vi "Find Structures.vi"(8 "error in (no error)":errorcluster, 9 "i in":i32, 11 "VI in":refnum<vi>) -> (0 "error out":errorcluster, 1 "i out":i32, 3 "Structures":T1[](array[typedef]))   [LabVIEW 2023, in "VIDoc Parsing.lvlib" / "Structure Reporter.lvlib"]
uses:
  Structure Reporter.lvlib
  Structure Result 2.ctl
  <vilib>/Utility/traverseref.llb/TRef TravTarget.ctl
  <vilib>/Utility/traverseref.llb/VI Scripting - Traverse.lvlib
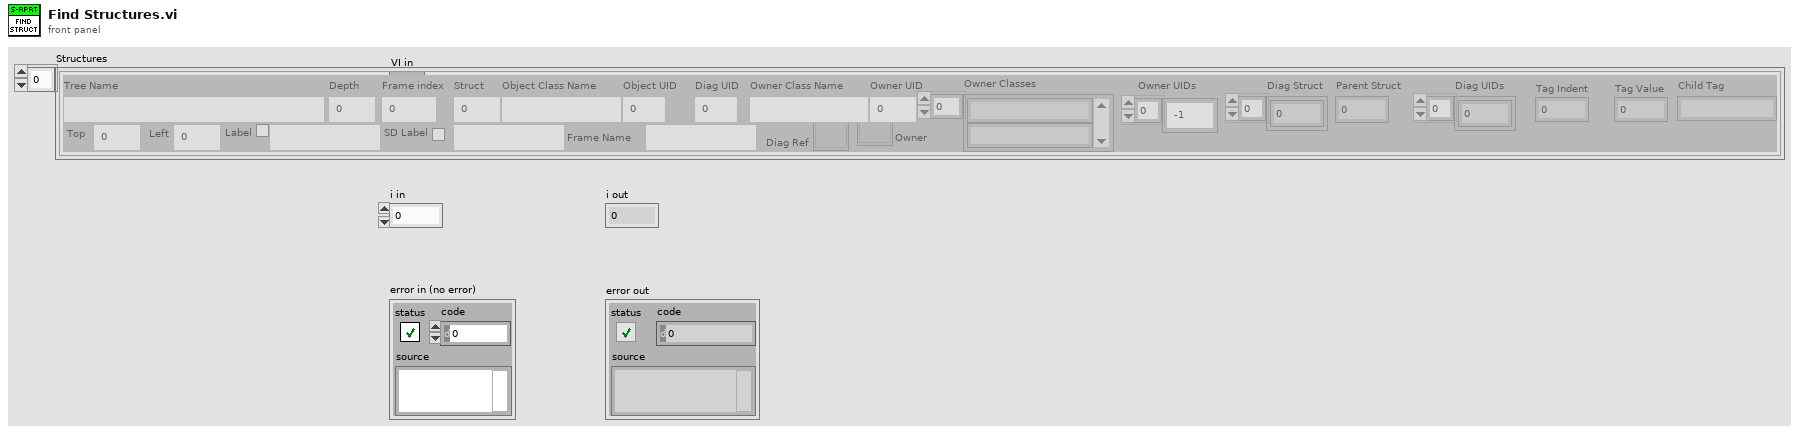
[diagram p1: front panel]
types:
  T1 = typedef "VIDoc Parsing.lvlib/Structure Reporter.lvlib/Structure Result 2.ctl" = cluster{"Depth":i32, "Top":i32, "Left":i32, "Frame index":i32, "Struct":i32, "Object Class Name":string, "Object UID":i32, "Label Visible":bool, "Object Label":string, "SD Label Visible":bool, "Object SD Label":string, "Frame Name":string, "Diag UID":i32, "Owner Class Name":string, "Owner UID":i32, "Diag Struct":i32[], "Parent Struct":i32, "Diag UIDs":i32[], "Tree Name":string, "Diag Ref":refnum<vi>, "Owner Classes":string[], "Owner":refnum<vi>, "Owner UIDs":i32[], "Tag Indent":i32, "Tag Value":i32, "Child Tag":string}
  T2 = typedef "TRef TravTarget.ctl" = enum16{"FP", "BD", "Other"}
  T3 = enum32{"Conditional Disable Style", "Diagram Disable Style", "Type Specialization Style"}
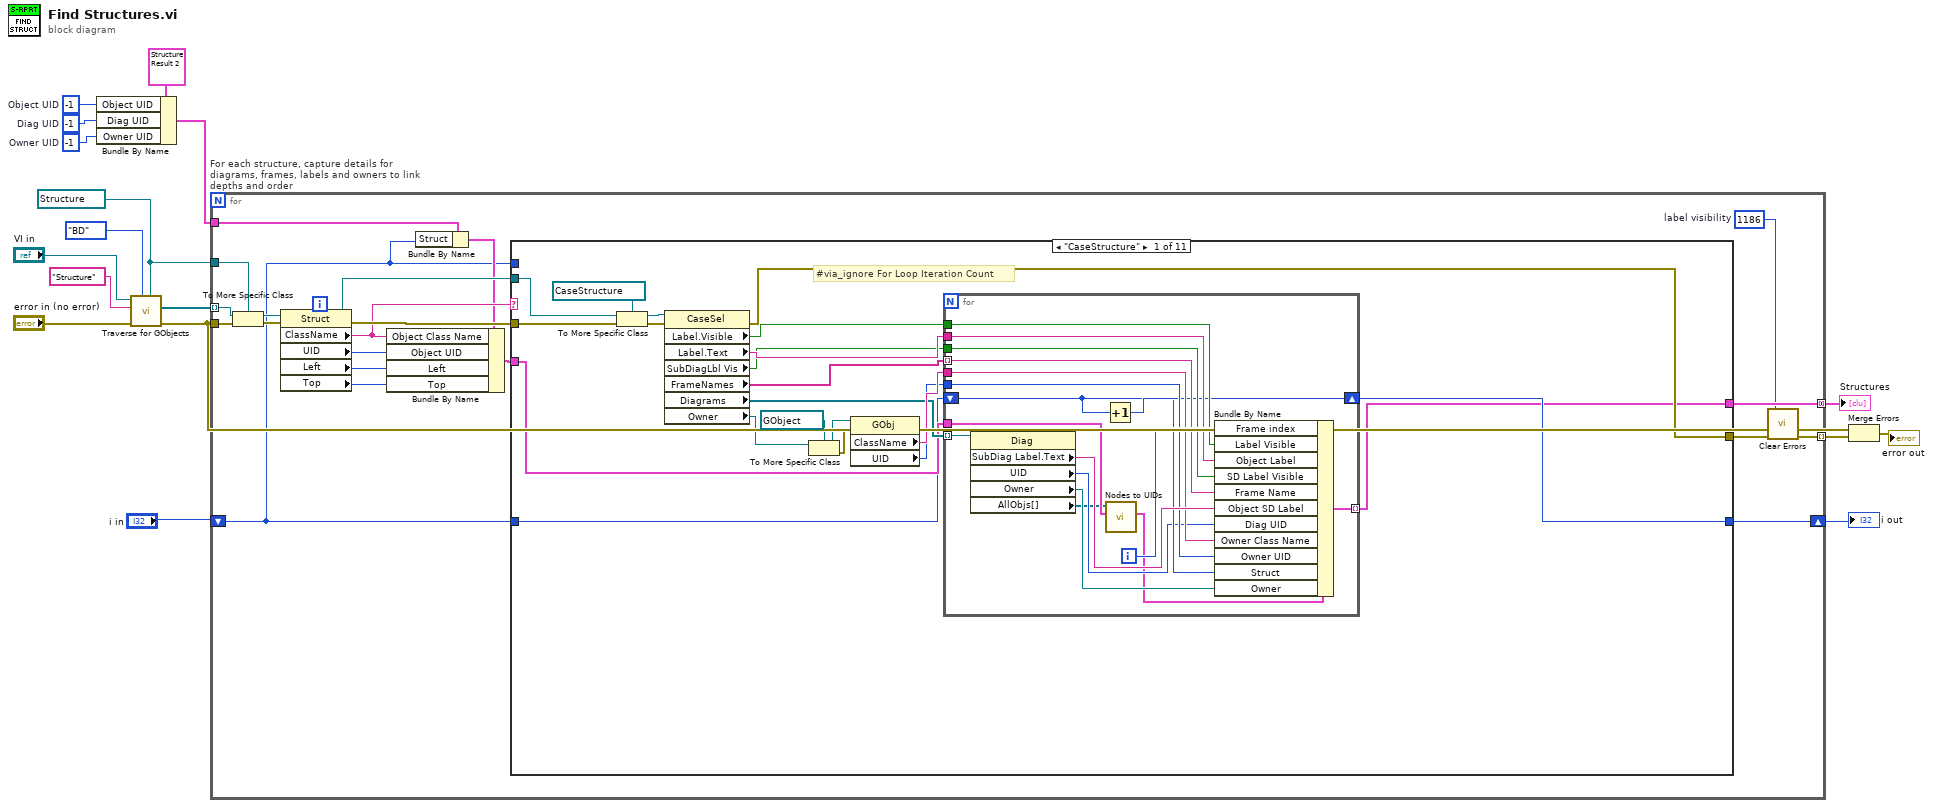
[diagram p0: block diagram]
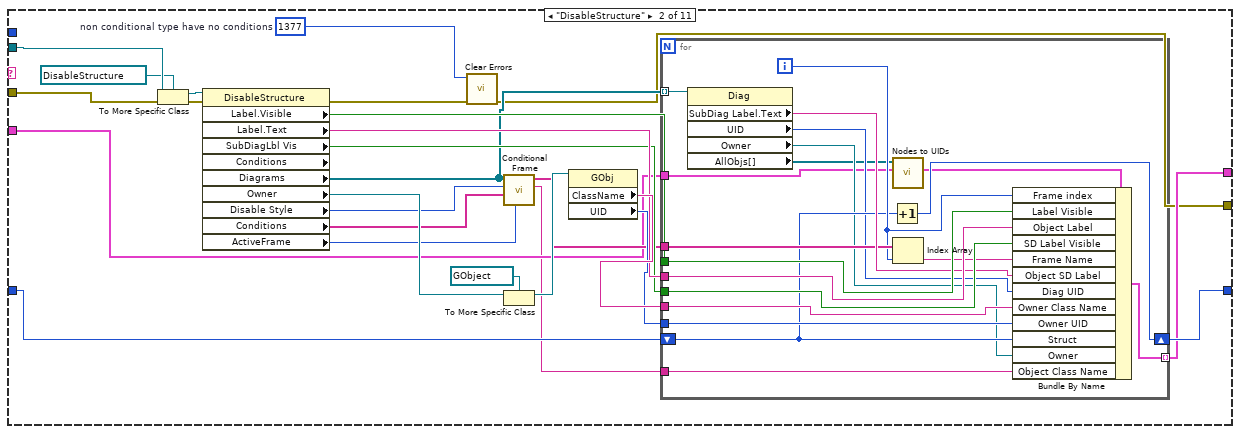
[diagram p2: hidden frame]
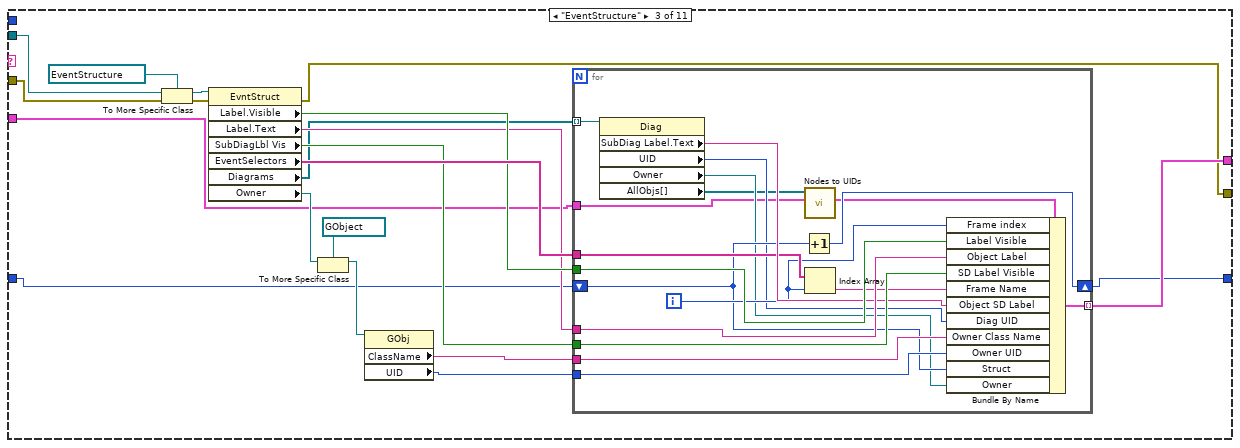
[diagram p3: hidden frame]
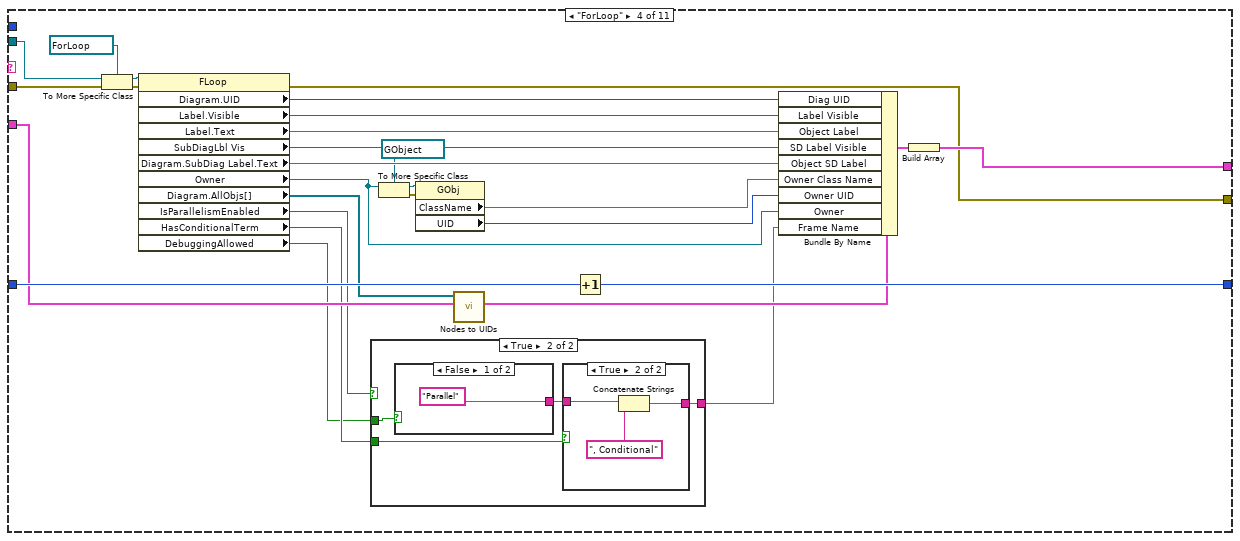
[diagram p4: hidden frame]
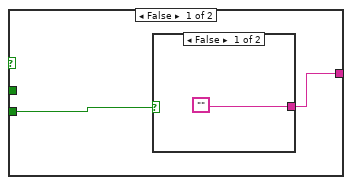
[diagram p5: hidden frame]
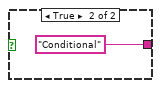
[diagram p6: hidden frame]
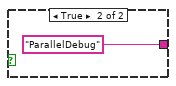
[diagram p8: hidden frame]
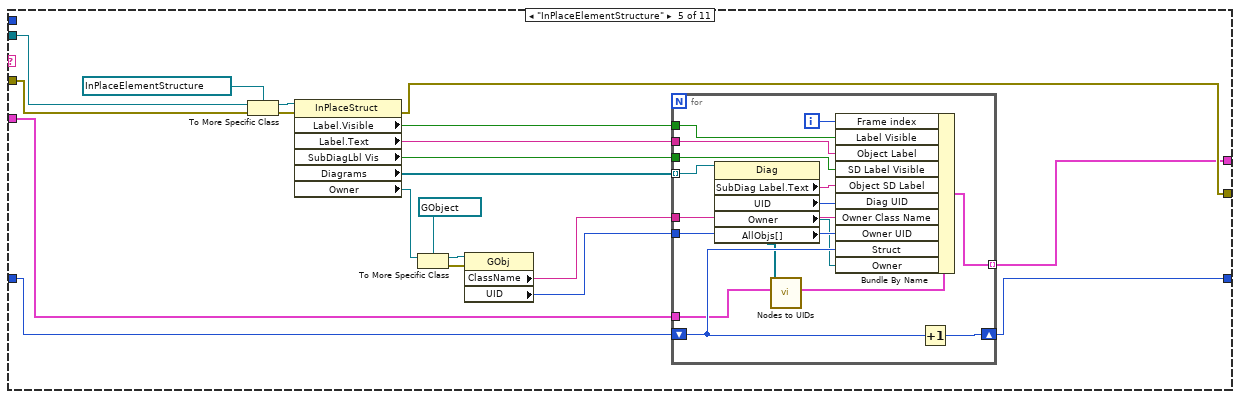
[diagram p9: hidden frame]
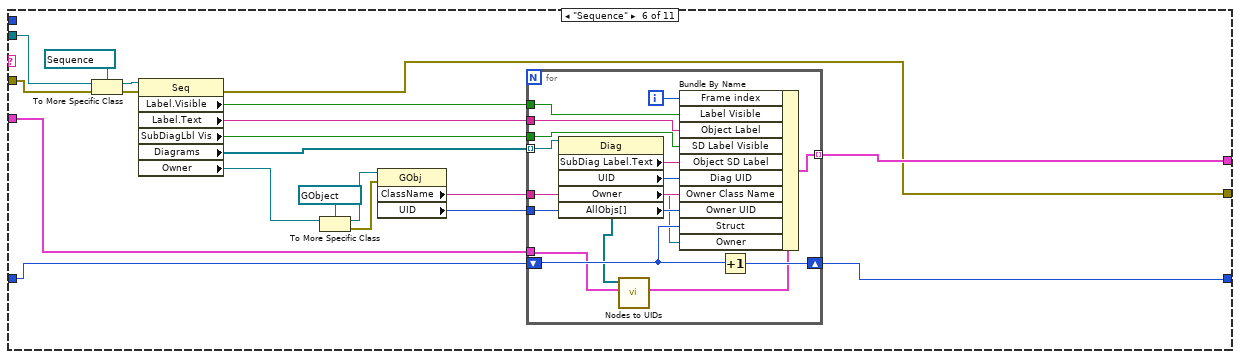
[diagram p10: hidden frame]
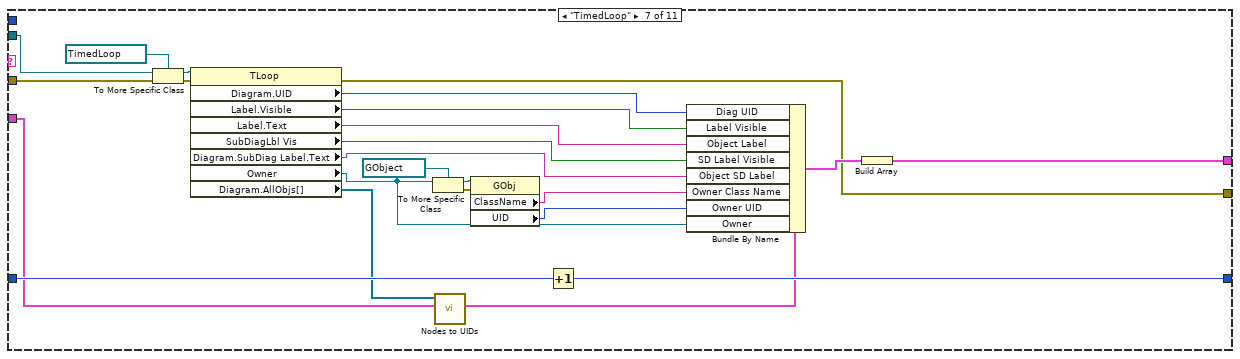
[diagram p11: hidden frame]
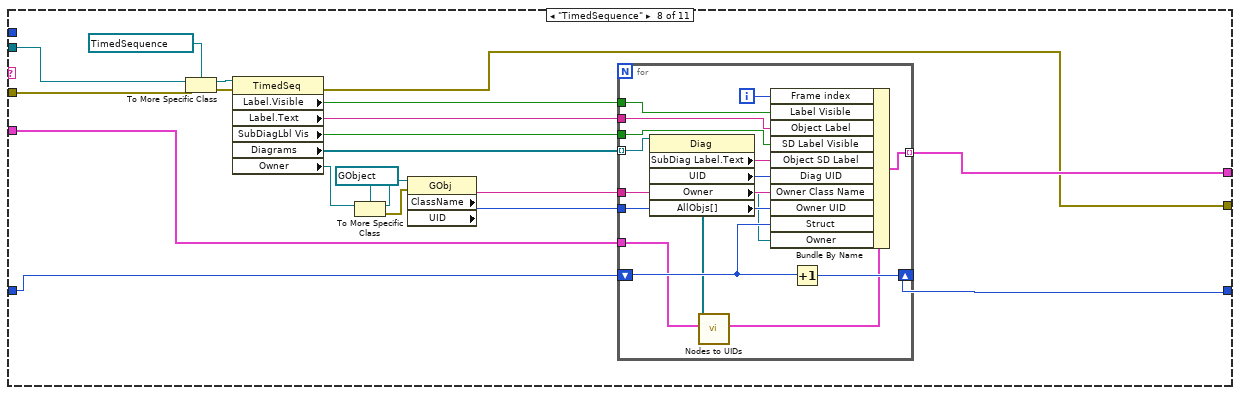
[diagram p12: hidden frame]
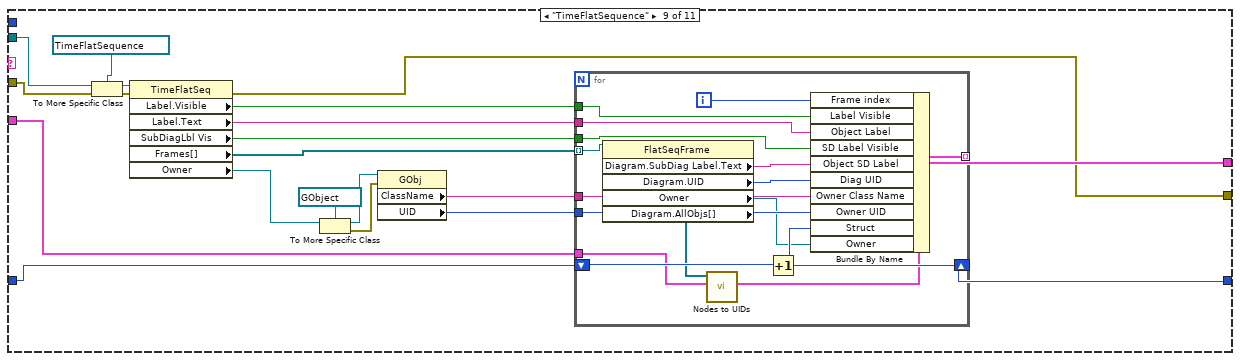
[diagram p13: hidden frame]
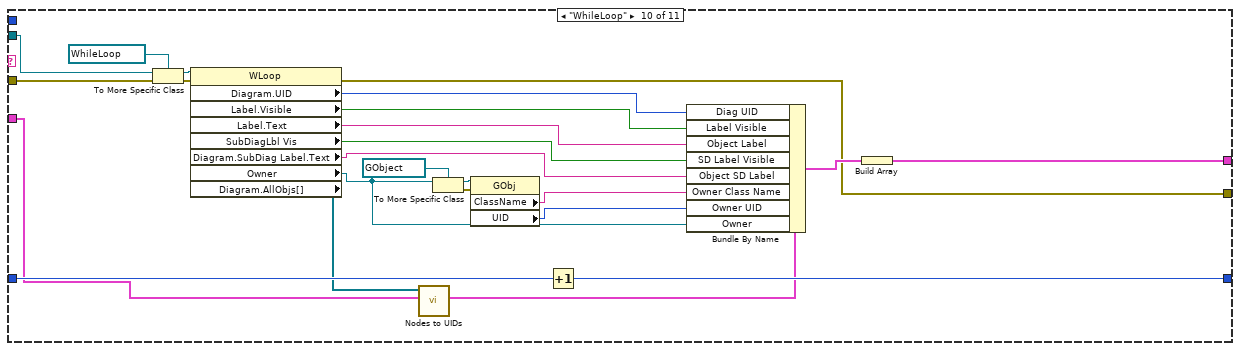
[diagram p14: hidden frame]
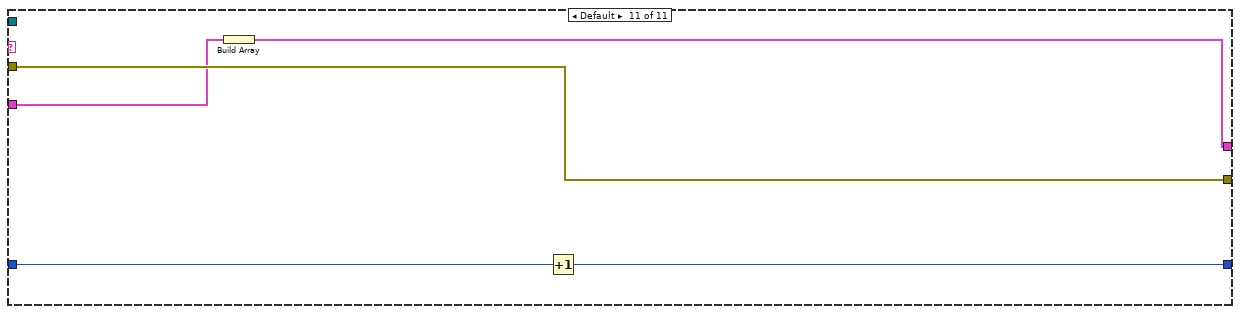
[diagram p15: hidden frame]
diagram:
  w3 = -1  # Owner UID
  w4 = -1  # Diag UID
  w5 = -1  # Object UID
  w15 = refnum<vi> refnum ("Other Refnum")
  n1 = Bundle By Name(cluster=T1 {"Depth"=0, "Top"=0, "Left"=0, "Frame index"=0, "Struct"=0, "Object Class Name"="", "Object UID"=0, "Label Visible"=FALSE, "Object Label"="", "SD Label Visible"=FALSE, "Object SD Label"="", "Frame Name"="", "Diag UID"=0, "Owner Class Name"="", "Owner UID"=0, "Diag Struct"=[], "Parent Struct"=0, "Diag UIDs"=[], "Tree Name"="", "Diag Ref"=refnum, "Owner Classes"=[], "Owner"=refnum, "Owner UIDs"=[], "Tag Indent"=0, "Tag Value"=0, "Child Tag"=""}, "Object UID"=w5, "Diag UID"=w4, "Owner UID"=w3) -> (w2:T1)
  n2 = call <vilib>:"Traverse for GObjects.vi"("Other Refnum"=w15, "Traverse Target"=TRef_TravTarget."BD", "error in (no error)"="error in (no error)", "Class Name"="Structure", "VI Refnum"="VI in") -> ("error out"=w1:errorcluster, "References"=w14:refnum<vi>[])  [unwired: 3 in, 2 out]
  n3 = for "For each structure, capture details for diagrams, frames, labels and owners to link depths and order" {
    tunnel: w14 -> [w37] mode=indexing
    tunnel: w15 -> [w36]
    tunnel: w1 -> [w34]
    tunnel: w2 -> [w23]
    tunnel: [w30] -> w16 mode=concatenating
    tunnel: [w19] -> w10 mode=indexing
    shift-right: [w20] -> w7
    shift-left: "i in" -> [w21]
    w18 = 1186  # label visibility
    n4 = To More Specific Class(target class=w36, reference=w37, error in=w34) -> (specific class reference=w35:refnum<vi>, error out=w33:errorcluster)
    n5 = property class="Struct"(reference=w35, error in=w33) -> (reference out=w32:refnum<vi>, error out=w31:errorcluster, "ClassName"=w24:string, "UID"=w29:i32, "Left"=w27:i32, "Top"=w26:i32)
    n6 = Bundle By Name(cluster=w23, "Struct"=w21) -> (w22:T1)
    n7 = Bundle By Name(cluster=w22, "Object Class Name"=w24, "Object UID"=w29, "Left"=w27, "Top"=w26) -> (w28:T1)
    n8 = case shown="\"CaseStructure\"" w24 {
      tunnel: w32 -> [w57 w100 w139 w164 w207 w255 w296 w302 w351 w392 _]
      tunnel: w31 -> [w56 w99 w138 w186 w206 w254 w295 w315 w350 w391 w396]
      tunnel: w28 -> [w42 w79 w123 w167 w201 w246 w275 w307 w343 w370 w393]
      tunnel: [w38 w84 w127 w162 w202 w242 w286 w300 w339 w382 w397] -> w30
      tunnel: w21 -> [_ _ _ _ _ _ _ _ _ _ _]
      tunnel: [w43 w77 w125 w161 w203 w240 w279 w299 w337 w375 w396] -> w25
      tunnel: [w39 w86 w121 w170 w205 w237 w277 w297 w334 w373 w394] -> w20
      tunnel: w21 -> [w40 w87 w122 w171 w204 w238 w278 w298 w335 w374 w395]
      frame "CaseStructure" {
        # "#via_ignore For Loop Iteration Count"
        n9 = To More Specific Class(target class=refnum<vi> refnum ("Other Refnum"), reference=w57, error in=w56) -> (specific class reference=w58:refnum<vi>, error out=w47:errorcluster)
        n10 = property class="CaseSel"(reference=w58, error in=w47) -> (error out=w43:errorcluster, "Label.Visible"=w53:bool, "Label.Text"=w46:string, "SubDiagLbl Vis"=w45:bool, "FrameNames"=w54:string[], "Diagrams"=w44:refnum<vi>[], "Owner"=w41:refnum<vi>)  [unwired: 1 out]
        n11 = To More Specific Class(target class=refnum<vi> refnum ("Other Refnum"), reference=w41) -> (specific class reference=w51:refnum<vi>, error out=w50:errorcluster)  [unwired: 1 in]
        n12 = property class="GObj"(reference=w51, error in=w50) -> ("ClassName"=w49:string, "UID"=w48:i32)  [unwired: 2 out]
        n13 = for {
          tunnel: w54 -> [w70] mode=indexing
          tunnel: w53 -> [w74]
          tunnel: w49 -> [w69]
          tunnel: w48 -> [w68]
          tunnel: w42 -> [w61]
          tunnel: w46 -> [w73]
          tunnel: w45 -> [w72]
          tunnel: [w67] -> w38 mode=indexing
          tunnel: w44 -> [w66] mode=indexing
          shift-right: [w65] -> w39
          shift-left: w40 -> [w64]
          i -> [w75]
          n14 = property class="Diag"(reference=w66) -> ("SubDiag Label.Text"=w71:string, "UID"=w63:i32, "Owner"=w62:refnum<vi>, "AllObjs[]"=w59:refnum<vi>[])  [unwired: 1 in, 2 out]
          n15 = Increment(x=w64) -> (x+1=w65:i32)
          n16 = call "Nodes to UIDs.vi"("cluster"=w61, "All Objects[]"=w59) -> ("Nodes"=w60:T1)  [unwired: 9 in]
          n17 = Bundle By Name(cluster=w60, "Frame index"=w75, "Label Visible"=w74, "Object Label"=w73, "SD Label Visible"=w72, "Frame Name"=w70, "Object SD Label"=w71, "Diag UID"=w63, "Owner Class Name"=w69, "Owner UID"=w68, "Struct"=w64, "Owner"=w62) -> (w67:T1)
        }
      }
      frame "DisableStructure" {
        w76 = 1377  # non conditional type have no conditions
        n18 = To More Specific Class(target class=refnum<vi> refnum ("Other Refnum"), reference=w100, error in=w99) -> (specific class reference=w101:refnum<vi>, error out=w92:errorcluster)
        n19 = property class="DisableStructure" props=["Label", "Visible", "Label", "Text", "SubDiagLbl Vis", "Conditions", "Diagrams", "Owner", "Disable Style", "Conditions", "ActiveFrame"](reference=w101, error in=w92) -> (error out=w89:errorcluster, "Label.Visible"=w97:bool, "Label.Text"=w91:string, "SubDiagLbl Vis"=w90:bool, "Diagrams"=w80:refnum<vi>[], "Owner"=w88:refnum<vi>, "Disable Style"=w85:T3, "Conditions"=w83:string[], "ActiveFrame"=w82:i16)  [unwired: 2 out]
        n20 = call <vilib>:"Clear Errors.vi"("error in (no error)"=w89, "specific error code to clear (0: all)"=w76) -> ("error out"=w77:errorcluster)  [unwired: 4 in, 1 out]
        n21 = call "Conditional Frame.vi"("ActiveFrame"=w82, "Conditions in"=w83, "Disable Style"=w85, "Diagrams"=w80) -> ("Class"=w78:string, "Conditions out"=w81:string[])  [unwired: 6 in]
        n22 = To More Specific Class(target class=refnum<vi> refnum ("Other Refnum"), reference=w88) -> (specific class reference=w95:refnum<vi>)  [unwired: 1 in, 1 out]
        n23 = property class="GObj"(reference=w95) -> ("ClassName"=w94:string, "UID"=w93:i32)  [unwired: 1 in, 2 out]
        n24 = for {
          tunnel: w81 -> [w112]
          tunnel: w97 -> [w120]
          tunnel: w94 -> [w116]
          tunnel: w93 -> [w115]
          tunnel: w79 -> [w104]
          tunnel: w91 -> [w119]
          tunnel: w90 -> [w118]
          tunnel: [w114] -> w84 mode=indexing
          tunnel: w80 -> [w113] mode=indexing
          shift-right: [w108] -> w86
          shift-left: w87 -> [w109]
          tunnel: w78 -> [w102]
          i -> [w111]
          n25 = property class="Diag"(reference=w113) -> ("SubDiag Label.Text"=w117:string, "UID"=w107:i32, "Owner"=w106:refnum<vi>, "AllObjs[]"=w105:refnum<vi>[])  [unwired: 1 in, 2 out]
          n26 = Increment(x=w109) -> (x+1=w108:i32)
          n27 = call "Nodes to UIDs.vi"("cluster"=w104, "All Objects[]"=w105) -> ("Nodes"=w103:T1)  [unwired: 9 in]
          n28 = Index Array(array=w112, index=w111) -> (element=w110:string)
          n29 = Bundle By Name(cluster=w103, "Frame index"=w111, "Label Visible"=w120, "Object Label"=w119, "SD Label Visible"=w118, "Frame Name"=w110, "Object SD Label"=w117, "Diag UID"=w107, "Owner Class Name"=w116, "Owner UID"=w115, "Struct"=w109, "Owner"=w106, "Object Class Name"=w102) -> (w114:T1)
        }
      }
      frame "EventStructure" {
        n30 = To More Specific Class(target class=refnum<vi> refnum ("Other Refnum"), reference=w139, error in=w138) -> (specific class reference=w140:refnum<vi>, error out=w130:errorcluster)
        n31 = property class="EvntStruct"(reference=w140, error in=w130) -> (error out=w125:errorcluster, "Label.Visible"=w135:bool, "Label.Text"=w129:string, "SubDiagLbl Vis"=w128:bool, "EventSelectors"=w136:string[], "Diagrams"=w126:refnum<vi>[], "Owner"=w124:refnum<vi>)  [unwired: 1 out]
        n32 = To More Specific Class(target class=refnum<vi> refnum ("Other Refnum"), reference=w124) -> (specific class reference=w133:refnum<vi>)  [unwired: 1 in, 1 out]
        n33 = property class="GObj"(reference=w133) -> ("ClassName"=w132:string, "UID"=w131:i32)  [unwired: 1 in, 2 out]
        n34 = for {
          tunnel: w136 -> [w150]
          tunnel: w135 -> [w158]
          tunnel: w132 -> [w154]
          tunnel: w131 -> [w153]
          tunnel: w123 -> [w142]
          tunnel: w129 -> [w157]
          tunnel: w128 -> [w156]
          tunnel: [w152] -> w127 mode=indexing
          tunnel: w126 -> [w151] mode=indexing
          shift-right: [w147] -> w121
          shift-left: w122 -> [w146]
          i -> [w149]
          n35 = property class="Diag"(reference=w151) -> ("SubDiag Label.Text"=w155:string, "UID"=w145:i32, "Owner"=w144:refnum<vi>, "AllObjs[]"=w143:refnum<vi>[])  [unwired: 1 in, 2 out]
          n36 = Increment(x=w146) -> (x+1=w147:i32)
          n37 = call "Nodes to UIDs.vi"("cluster"=w142, "All Objects[]"=w143) -> ("Nodes"=w141:T1)  [unwired: 9 in]
          n38 = Index Array(array=w150, index=w149) -> (element=w148:string)
          n39 = Bundle By Name(cluster=w141, "Frame index"=w149, "Label Visible"=w158, "Object Label"=w157, "SD Label Visible"=w156, "Frame Name"=w148, "Object SD Label"=w155, "Diag UID"=w145, "Owner Class Name"=w154, "Owner UID"=w153, "Struct"=w146, "Owner"=w144) -> (w152:T1)
        }
      }
      frame "ForLoop" {
        n40 = To More Specific Class(target class=refnum<vi> refnum ("Other Refnum"), reference=w164, error in=w186) -> (specific class reference=w184:refnum<vi>, error out=w183:errorcluster)
        n41 = property class="FLoop"(reference=w184, error in=w183) -> (error out=w161:errorcluster, "Diagram.UID"=w172:i32, "Label.Visible"=w182:bool, "Label.Text"=w181:string, "SubDiagLbl Vis"=w180:bool, "Diagram.SubDiag Label.Text"=w179:string, "Owner"=w169:refnum<vi>, "Diagram.AllObjs[]"=w168:refnum<vi>[], "IsParallelismEnabled"=w159:bool, "HasConditionalTerm"=w165:bool, "DebuggingAllowed"=w163:bool)  [unwired: 1 out]
        n42 = case shown="True" w159 {
          tunnel: w165 -> [w188 w193]
          tunnel: w163 -> [_ w194]
          tunnel: [w187 w191] -> w160
          frame False {
            n43 = case shown="False" w188 {
              tunnel: ["" "Conditional"] -> w187
              frame False {
              }
              frame True {
              }
            }
          }
          frame True {
            n44 = case shown="False" w194 {
              tunnel: ["Parallel" "ParallelDebug"] -> w192
              frame False {
              }
              frame True {
              }
            }
            n45 = case shown="True" w193 {
              tunnel: w192 -> [w195 w198]
              tunnel: [w195 w197] -> w191
              frame False {
              }
              frame True {
                n46 = Concatenate Strings(w198, ", Conditional") -> (w197:string)
              }
            }
          }
        }
        n47 = To More Specific Class(target class=refnum<vi> refnum ("Other Refnum"), reference=w169) -> (specific class reference=w177:refnum<vi>, error out=w176:errorcluster)  [unwired: 1 in]
        n48 = property class="GObj"(reference=w177, error in=w176) -> ("ClassName"=w174:string, "UID"=w173:i32)  [unwired: 2 out]
        n49 = call "Nodes to UIDs.vi"("cluster"=w167, "All Objects[]"=w168) -> ("Nodes"=w166:T1)  [unwired: 9 in]
        n50 = Increment(x=w171) -> (x+1=w170:i32)
        n51 = Bundle By Name(cluster=w166, "Diag UID"=w172, "Label Visible"=w182, "Object Label"=w181, "SD Label Visible"=w180, "Object SD Label"=w179, "Owner Class Name"=w174, "Owner UID"=w173, "Owner"=w169, "Frame Name"=w160) -> (w178:T1)
        n52 = Build Array(w178) -> (w162:T1[])
      }
      frame "InPlaceElementStructure" {
        n53 = To More Specific Class(target class=refnum<vi> refnum ("Other Refnum"), reference=w207, error in=w206) -> (specific class reference=w220:refnum<vi>, error out=w212:errorcluster)
        n54 = property class="InPlaceStruct"(reference=w220, error in=w212) -> (error out=w203:errorcluster, "Label.Visible"=w218:bool, "Label.Text"=w211:string, "SubDiagLbl Vis"=w210:bool, "Diagrams"=w209:refnum<vi>[], "Owner"=w208:refnum<vi>)  [unwired: 1 out]
        n55 = To More Specific Class(target class=refnum<vi> refnum ("Other Refnum"), reference=w208) -> (specific class reference=w216:refnum<vi>, error out=w215:errorcluster)  [unwired: 1 in]
        n56 = property class="GObj"(reference=w216, error in=w215) -> ("ClassName"=w214:string, "UID"=w213:i32)  [unwired: 2 out]
        n57 = for {
          tunnel: w218 -> [w235]
          tunnel: w214 -> [w231]
          tunnel: w213 -> [w230]
          tunnel: w201 -> [w221]
          tunnel: w211 -> [w234]
          tunnel: w210 -> [w233]
          tunnel: [w229] -> w202 mode=indexing
          tunnel: w209 -> [w228] mode=indexing
          shift-right: [w227] -> w205
          shift-left: w204 -> [w226]
          i -> [w236]
          n58 = property class="Diag"(reference=w228) -> ("SubDiag Label.Text"=w232:string, "UID"=w225:i32, "Owner"=w224:refnum<vi>, "AllObjs[]"=w223:refnum<vi>[])  [unwired: 1 in, 2 out]
          n59 = call "Nodes to UIDs.vi"("cluster"=w221, "All Objects[]"=w223) -> ("Nodes"=w222:T1)  [unwired: 9 in]
          n60 = Bundle By Name(cluster=w222, "Frame index"=w236, "Label Visible"=w235, "Object Label"=w234, "SD Label Visible"=w233, "Object SD Label"=w232, "Diag UID"=w225, "Owner Class Name"=w231, "Owner UID"=w230, "Struct"=w226, "Owner"=w224) -> (w229:T1)
          n61 = Increment(x=w226) -> (x+1=w227:i32)
        }
      }
      frame "Sequence" {
        n62 = To More Specific Class(target class=refnum<vi> refnum ("Other Refnum"), reference=w255, error in=w254) -> (specific class reference=w256:refnum<vi>, error out=w245:errorcluster)
        n63 = property class="Seq"(reference=w256, error in=w245) -> (error out=w240:errorcluster, "Label.Visible"=w252:bool, "Label.Text"=w244:string, "SubDiagLbl Vis"=w243:bool, "Diagrams"=w241:refnum<vi>[], "Owner"=w239:refnum<vi>)  [unwired: 1 out]
        n64 = To More Specific Class(target class=refnum<vi> refnum ("Other Refnum"), reference=w239) -> (specific class reference=w250:refnum<vi>, error out=w249:errorcluster)  [unwired: 1 in]
        n65 = property class="GObj"(reference=w250, error in=w249) -> ("ClassName"=w248:string, "UID"=w247:i32)  [unwired: 2 out]
        n66 = for {
          tunnel: w252 -> [w271]
          tunnel: w248 -> [w267]
          tunnel: w247 -> [w266]
          tunnel: w246 -> [w258]
          tunnel: w244 -> [w270]
          tunnel: w243 -> [w269]
          tunnel: [w265] -> w242 mode=indexing
          tunnel: w241 -> [w264] mode=indexing
          shift-right: [w263] -> w237
          shift-left: w238 -> [w262]
          i -> [w272]
          n67 = property class="Diag"(reference=w264) -> ("SubDiag Label.Text"=w268:string, "UID"=w261:i32, "Owner"=w260:refnum<vi>, "AllObjs[]"=w259:refnum<vi>[])  [unwired: 1 in, 2 out]
          n68 = call "Nodes to UIDs.vi"("cluster"=w258, "All Objects[]"=w259) -> ("Nodes"=w257:T1)  [unwired: 9 in]
          n69 = Bundle By Name(cluster=w257, "Frame index"=w272, "Label Visible"=w271, "Object Label"=w270, "SD Label Visible"=w269, "Object SD Label"=w268, "Diag UID"=w261, "Owner Class Name"=w267, "Owner UID"=w266, "Struct"=w262, "Owner"=w260) -> (w265:T1)
          n70 = Increment(x=w262) -> (x+1=w263:i32)
        }
      }
      frame "TimedLoop" {
        n71 = To More Specific Class(target class=refnum<vi> refnum ("Other Refnum"), reference=w296, error in=w295) -> (specific class reference=w293:refnum<vi>, error out=w292:errorcluster)
        n72 = property class="TLoop"(reference=w293, error in=w292) -> (error out=w279:errorcluster, "Diagram.UID"=w280:i32, "Label.Visible"=w291:bool, "Label.Text"=w290:string, "SubDiagLbl Vis"=w289:bool, "Diagram.SubDiag Label.Text"=w288:string, "Owner"=w276:refnum<vi>, "Diagram.AllObjs[]"=w274:refnum<vi>[])  [unwired: 1 out]
        n73 = To More Specific Class(target class=refnum<vi> refnum ("Other Refnum"), reference=w276) -> (specific class reference=w285:refnum<vi>, error out=w284:errorcluster)  [unwired: 1 in]
        n74 = call "Nodes to UIDs.vi"("cluster"=w275, "All Objects[]"=w274) -> ("Nodes"=w273:T1)  [unwired: 9 in]
        n75 = property class="GObj"(reference=w285, error in=w284) -> ("ClassName"=w282:string, "UID"=w281:i32)  [unwired: 2 out]
        n76 = Increment(x=w278) -> (x+1=w277:i32)
        n77 = Bundle By Name(cluster=w273, "Diag UID"=w280, "Label Visible"=w291, "Object Label"=w290, "SD Label Visible"=w289, "Object SD Label"=w288, "Owner Class Name"=w282, "Owner UID"=w281, "Owner"=w276) -> (w287:T1)
        n78 = Build Array(w287) -> (w286:T1[])
      }
      frame "TimedSequence" {
        n79 = To More Specific Class(target class=refnum<vi> refnum ("Other Refnum"), reference=w302, error in=w315) -> (specific class reference=w316:refnum<vi>, error out=w306:errorcluster)
        n80 = property class="TimedSeq"(reference=w316, error in=w306) -> (error out=w299:errorcluster, "Label.Visible"=w313:bool, "Label.Text"=w305:string, "SubDiagLbl Vis"=w304:bool, "Diagrams"=w303:refnum<vi>[], "Owner"=w301:refnum<vi>)  [unwired: 1 out]
        n81 = To More Specific Class(target class=refnum<vi> refnum ("Other Refnum"), reference=w301) -> (specific class reference=w311:refnum<vi>, error out=w310:errorcluster)  [unwired: 1 in]
        n82 = property class="GObj"(reference=w311, error in=w310) -> ("ClassName"=w309:string, "UID"=w308:i32)  [unwired: 2 out]
        n83 = for {
          tunnel: w313 -> [w331]
          tunnel: w309 -> [w327]
          tunnel: w308 -> [w326]
          tunnel: w307 -> [w318]
          tunnel: w305 -> [w330]
          tunnel: w304 -> [w329]
          tunnel: [w325] -> w300 mode=indexing
          tunnel: w303 -> [w324] mode=indexing
          shift-right: [w323] -> w297
          shift-left: w298 -> [w322]
          i -> [w332]
          n84 = property class="Diag"(reference=w324) -> ("SubDiag Label.Text"=w328:string, "UID"=w321:i32, "Owner"=w320:refnum<vi>, "AllObjs[]"=w319:refnum<vi>[])  [unwired: 1 in, 2 out]
          n85 = call "Nodes to UIDs.vi"("cluster"=w318, "All Objects[]"=w319) -> ("Nodes"=w317:T1)  [unwired: 9 in]
          n86 = Bundle By Name(cluster=w317, "Frame index"=w332, "Label Visible"=w331, "Object Label"=w330, "SD Label Visible"=w329, "Object SD Label"=w328, "Diag UID"=w321, "Owner Class Name"=w327, "Owner UID"=w326, "Struct"=w322, "Owner"=w320) -> (w325:T1)
          n87 = Increment(x=w322) -> (x+1=w323:i32)
        }
      }
      frame "TimeFlatSequence" {
        n88 = To More Specific Class(target class=refnum<vi> refnum ("Other Refnum"), reference=w351, error in=w350) -> (specific class reference=w352:refnum<vi>, error out=w342:errorcluster)
        n89 = property class="TimeFlatSeq"(reference=w352, error in=w342) -> (error out=w337:errorcluster, "Label.Visible"=w349:bool, "Label.Text"=w341:string, "SubDiagLbl Vis"=w340:bool, "Frames[]"=w338:refnum<vi>[], "Owner"=w336:refnum<vi>)  [unwired: 1 out]
        n90 = To More Specific Class(target class=refnum<vi> refnum ("Other Refnum"), reference=w336) -> (specific class reference=w347:refnum<vi>, error out=w346:errorcluster)  [unwired: 1 in]
        n91 = property class="GObj"(reference=w347, error in=w346) -> ("ClassName"=w345:string, "UID"=w344:i32)  [unwired: 2 out]
        n92 = for {
          tunnel: w349 -> [w367]
          tunnel: w345 -> [w363]
          tunnel: w344 -> [w362]
          tunnel: w343 -> [w355]
          tunnel: w341 -> [w366]
          tunnel: w340 -> [w365]
          tunnel: [w361] -> w339 mode=indexing
          tunnel: w338 -> [w360] mode=indexing
          shift-right: [w359] -> w334
          shift-left: w335 -> [w358]
          i -> [w368]
          n93 = property class="FlatSeqFrame"(reference=w360) -> ("Diagram.SubDiag Label.Text"=w364:string, "Diagram.UID"=w357:i32, "Owner"=w356:refnum<vi>, "Diagram.AllObjs[]"=w353:refnum<vi>[])  [unwired: 1 in, 2 out]
          n94 = call "Nodes to UIDs.vi"("cluster"=w355, "All Objects[]"=w353) -> ("Nodes"=w354:T1)  [unwired: 9 in]
          n95 = Increment(x=w358) -> (x+1=w359:i32)
          n96 = Bundle By Name(cluster=w354, "Frame index"=w368, "Label Visible"=w367, "Object Label"=w366, "SD Label Visible"=w365, "Object SD Label"=w364, "Diag UID"=w357, "Owner Class Name"=w363, "Owner UID"=w362, "Struct"=w358, "Owner"=w356) -> (w361:T1)
        }
      }
      frame "WhileLoop" {
        n97 = To More Specific Class(target class=refnum<vi> refnum ("Other Refnum"), reference=w392, error in=w391) -> (specific class reference=w389:refnum<vi>, error out=w388:errorcluster)
        n98 = property class="WLoop"(reference=w389, error in=w388) -> (error out=w375:errorcluster, "Diagram.UID"=w376:i32, "Label.Visible"=w387:bool, "Label.Text"=w386:string, "SubDiagLbl Vis"=w385:bool, "Diagram.SubDiag Label.Text"=w384:string, "Owner"=w372:refnum<vi>, "Diagram.AllObjs[]"=w371:refnum<vi>[])  [unwired: 1 out]
        n99 = call "Nodes to UIDs.vi"("cluster"=w370, "All Objects[]"=w371) -> ("Nodes"=w369:T1)  [unwired: 9 in]
        n100 = To More Specific Class(target class=refnum<vi> refnum ("Other Refnum"), reference=w372) -> (specific class reference=w381:refnum<vi>, error out=w380:errorcluster)  [unwired: 1 in]
        n101 = property class="GObj"(reference=w381, error in=w380) -> ("ClassName"=w378:string, "UID"=w377:i32)  [unwired: 2 out]
        n102 = Increment(x=w374) -> (x+1=w373:i32)
        n103 = Bundle By Name(cluster=w369, "Diag UID"=w376, "Label Visible"=w387, "Object Label"=w386, "SD Label Visible"=w385, "Object SD Label"=w384, "Owner Class Name"=w378, "Owner UID"=w377, "Owner"=w372) -> (w383:T1)
        n104 = Build Array(w383) -> (w382:T1[])
      }
      frame Default {
        n105 = Build Array(w393) -> (w397:T1[])
        n106 = Increment(x=w395) -> (x+1=w394:i32)
      }
    }
    n107 = call <vilib>:"Clear Errors.vi"("error in (no error)"=w25, "specific error code to clear (0: all)"=w18) -> ("error out"=w19:errorcluster)  [unwired: 4 in, 1 out]
  }
  "Structures" <- w16
  "i out" <- w7
  n108 = Merge Errors(w1, w10) -> (→"error out":errorcluster)
